vi "R-Series IO.vi"() -> ()   [LabVIEW 2010]
uses:
  <vilib>/eio/EIONode/EIONode.xnode
  <vilib>/rvi/eio/nirviEIOImplementation/nirviEIOImplementation.xnode
  <vilib>/rvi/eio/common/nirviEmuClasses.ctl
  <vilib>/rvi/eio/common/nirviEmuTemplateMethod_noerrors.vi
panel:
  out "Simulated Digital Port In (Raw)":u8
  out "Simulated Digital Port In (Boolean)":bool[](array[boolean])
  out "Simulated Analog In":i16
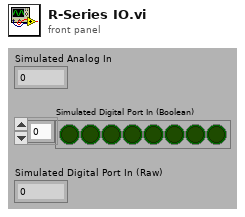
[diagram p1: front panel]
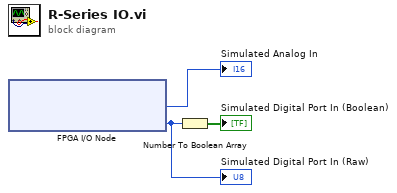
[diagram p0: block diagram]
diagram:
  n1 = xnode "FPGA I/O Node"() -> ("Simulated Analog In"=→"Simulated Analog In":i16, "Simulated Digital Port In"=w3:u8)  [unwired: 2 in, 2 out]
  "Simulated Digital Port In (Raw)" <- w3
  n2 = Number To Boolean Array(number=w3) -> (Boolean array=→"Simulated Digital Port In (Boolean)":bool[])
